vi "Timestamp File.vi"(8 "error in (no error)":errorcluster, 9 "Field name":string="File time stamp", 10 "Time Stamp":timestamp, 11 "File in":refnum<class "File.lvclass">) -> (0 "error out":errorcluster, 3 "File out":refnum<class "File.lvclass">)   [LabVIEW 2021, in "File.lvclass"]
uses:
  File.lvclass
  File.lvclass/File.ctl
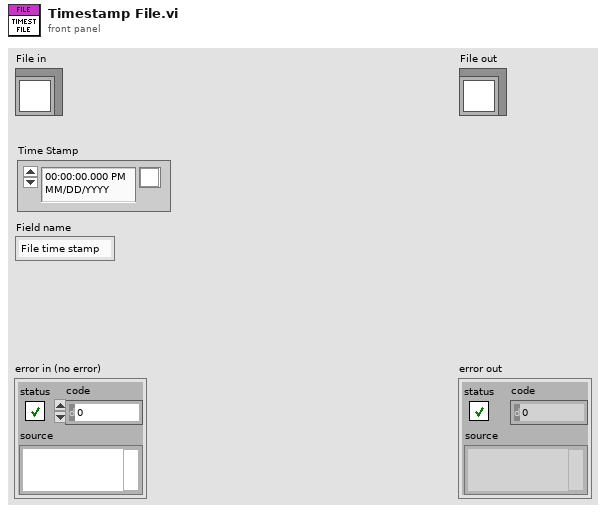
[diagram p1: front panel]
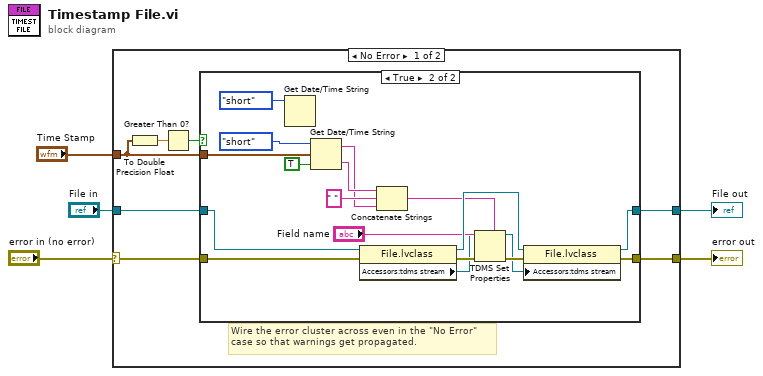
[diagram p0: block diagram]
diagram:
  n1 = case shown="No Error" "error in (no error)" {
    selector: "error in (no error)" -> [w9 w34]
    tunnel: [w6 w34] -> w4
    tunnel: [w8 w33] -> w2
    tunnel: "File in" -> [w7 w33]
    tunnel: "Time Stamp" -> [w10 _]
    frame No Error {
      # "Wire the error cluster across even in the \"No Error\"\ncase so that warnings get propagated."
      n2 = To Double Precision Float(number=w10) -> (double precision float=w12:dbl)
      n3 = Greater Than 0?(x=w12) -> (x > 0?=w11:bool)
      n4 = case shown="True" w11 {
        tunnel: w10 -> [_ w26]
        tunnel: w7 -> [w14 w25]
        tunnel: w9 -> [w13 w24]
        tunnel: [w14 w17] -> w8
        tunnel: [w13 w16] -> w6
        frame False {
        }
        frame True {
          n5 = Get Date/Time String(date format (0)=enum16{"short", "long", "abbreviated"}."short") -> ()  [unwired: 2 in, 2 out]
          n6 = Get Date/Time String(date format (0)=enum16{"short", "long", "abbreviated"}."short", seconds (now)=w26, want seconds? (F)=TRUE) -> (date string=w27:string, time string=w28:string)
          n7 = property class="File.lvclass"(reference=w25, error in=w24) -> (reference out=w23:refnum<class "File.lvclass">, error out=w20:errorcluster, "Accessors:tdms stream"=w15:refnum<k34>)
          n8 = Concatenate Strings(w28, " " ("string"), w27) -> (w21:string)
          n9 = TDMS Set Properties(5:w21, 7:"Field name", 8:w20, 11:w15) -> (0:w19:errorcluster, 3:w18:refnum<k34>)  [unwired: 2 in, 2 out]
          n10 = property class="File.lvclass"(reference=w23, error in=w19, "Accessors:tdms stream"=w18) -> (reference out=w17:refnum<class "File.lvclass">, error out=w16:errorcluster)
        }
      }
    }
    frame Error {
    }
  }
  "error out" <- w4
  "File out" <- w2
